vi "Core Actor (ROOT) - Dispatch Message to Child (Nested_Actor).vi"(8 "error in (no error)":errorcluster, 11 "Message_Distributor_Class in":refnum<class "Message_Distributor_Class.lvclass">) -> (0 "error out":errorcluster, 3 "Message_Distributor_Class out":refnum<class "Message_Distributor_Class.lvclass">)   [LabVIEW 2023, in "Actor_Message_Distributor.lvlib" / "Message_Distributor_Class.lvclass"]
uses:
  Message_Distributor_Class.lvclass
  Distributor - Ctrl - Trigger Event Cluster.ctl
  Usr Ev/Distributor - Ctrl - Enum - Events.ctl
  Message_Distributor_Class.lvclass/Message_Distributor_Class.ctl
  Message_Distributor_Class Messages/Core Actor - Send Actor Message Msg/Core Actor - Send Actor Message Msg.lvclass/Core Actor - Send Actor Message Msg.ctl
  <vilib>/ActorFramework/Message Enqueuer/Message Enqueuer.lvclass/Message Enqueuer.ctl
  <vilib>/ActorFramework/Message Enqueuer/Enqueue.vi
  Message_Distributor_Class Messages/Core Actor - Send Actor Message Msg/Core Actor - Send Actor Message Msg.lvclass
  C:/Program Files/National Instruments/LabVIEW 2023/vi.lib/ActorFramework/Message/Message.lvclass
  <vilib>/ActorFramework/Message Priority Queue/Priority Enqueue.vi
panel:
  out "Parent Trigger Event Cluster":T1
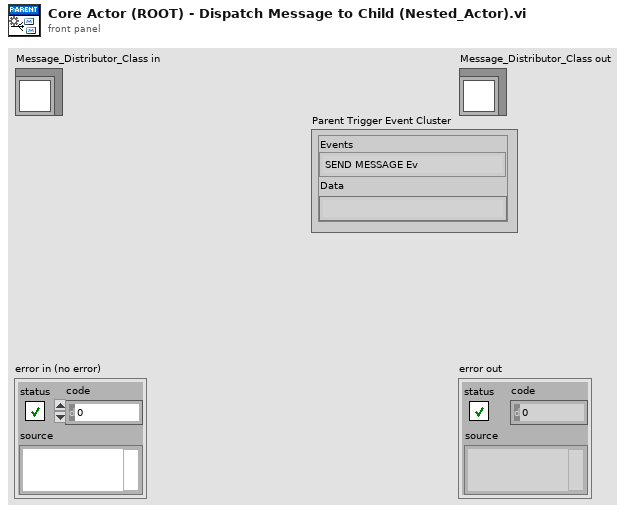
[diagram p1: front panel]
types:
  T1 = typedef "Actor_Message_Distributor.lvlib/Message_Distributor_Class.lvclass/Distributor - Ctrl - Trigger Event Cluster.ctl" = cluster{"Events":T2, "Data":string}
  T2 = typedef "Actor_Message_Distributor.lvlib/Message_Distributor_Class.lvclass/Distributor - Ctrl - Enum - Events.ctl" = enum16{"SEND MESSAGE Ev", "STOP_ACTOR Ev", "INIT_ACTOR Ev", "START Ev", "STOP Ev", "GET Ev", "SET Ev", "ERROR_HANDLER Ev", "RESET Ev", "DISPATCH MESSAGE 2 CHILDS Ev", "ECU RESET Ev"}
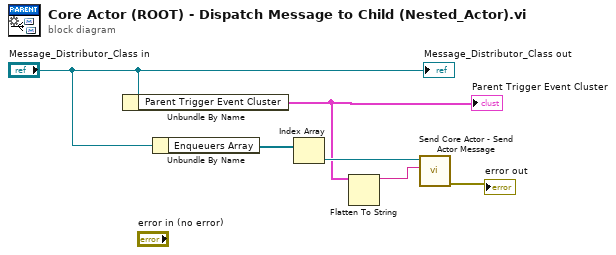
[diagram p0: block diagram]
diagram:
  n1 = Unbundle By Name("Message_Distributor_Class in") -> ("Parent Trigger Event Cluster"=w3:T1)
  "Parent Trigger Event Cluster" <- w3
  n2 = Unbundle By Name("Message_Distributor_Class in") -> ("Enqueuers Array"=w5:refnum<class "Message Enqueuer.lvclass">[])
  n3 = Index Array(array=w5) -> (element=w4:refnum<class "Message Enqueuer.lvclass">)  [unwired: 1 in]
  n4 = Flatten To String(anything=w3) -> (data string=w2:string)  [unwired: 3 in, 2 out]
  n5 = call "Send Core Actor - Send Actor Message.vi"("Value"=w2, "Message Enqueuer"=w4) -> ("error out"=→"error out":errorcluster)  [unwired: 8 in, 1 out]
  "Message_Distributor_Class out" <- "Message_Distributor_Class in"
